vi "Result.Numeric, Compare Value to Limits.vi"(8 "UL":dbl, 9 "LL":dbl, 10 "Value":dbl, 11 "LimType":T2) -> (1 "Desc":string, 3 "Status":T1=3 items=["LOG", "PASS", "FAIL", "ERROR"])   [LabVIEW 2019]
uses:
  Result.Limit Type.ctl
  Result.Measurement and Attribute Item Status.ctl
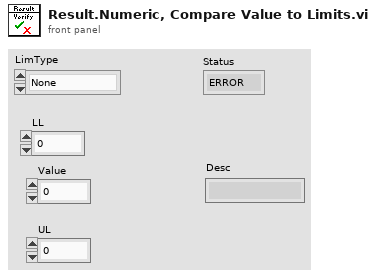
[diagram p1: front panel]
types:
  T1 = typedef "Result.Measurement and Attribute Item Status.ctl" = i32
  T2 = typedef "Result.Limit Type.ctl" = enum16{"None", "EQ", "NE", "GT", "LT", "GE", "LE", "GTLT", "GELE", "GELT", "GTLE", "LTGT", "LEGE", "LEGT", "LTGE", "Contains", "NotContains"}
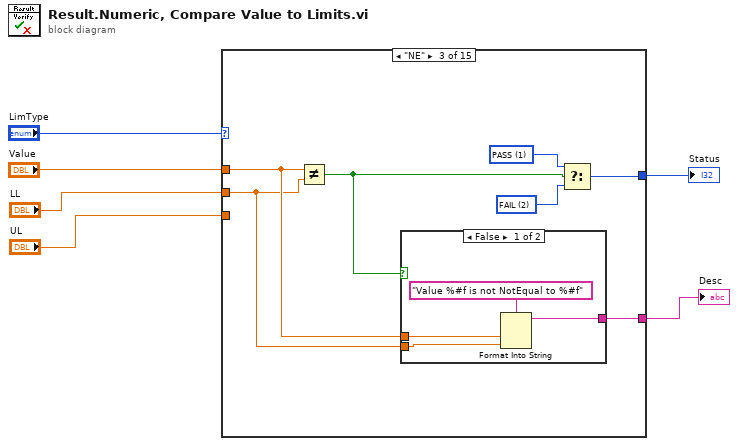
[diagram p0: block diagram]
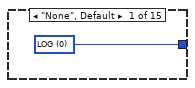
[diagram p2: hidden frame]
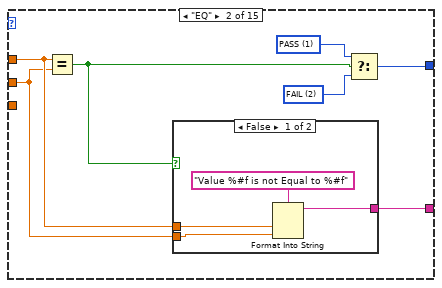
[diagram p3: hidden frame]
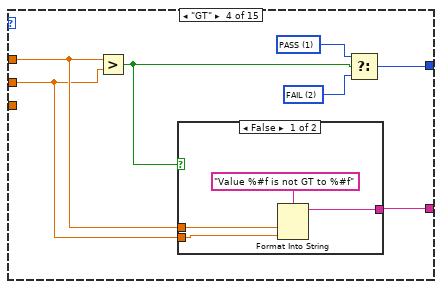
[diagram p6: hidden frame]
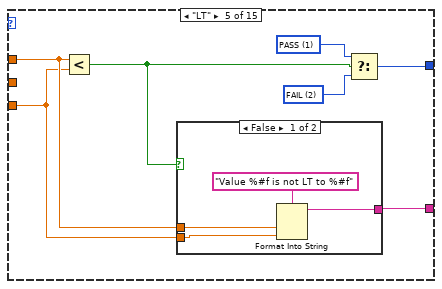
[diagram p8: hidden frame]
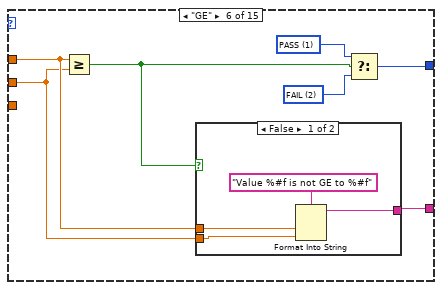
[diagram p10: hidden frame]
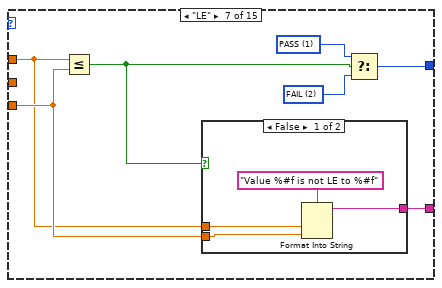
[diagram p12: hidden frame]
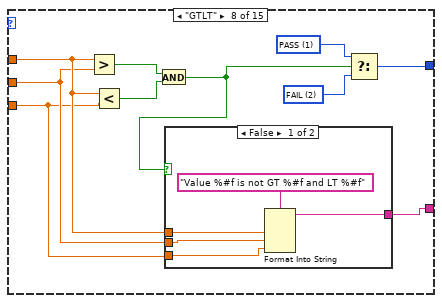
[diagram p14: hidden frame]
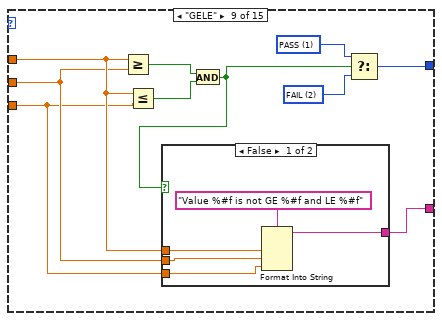
[diagram p16: hidden frame]
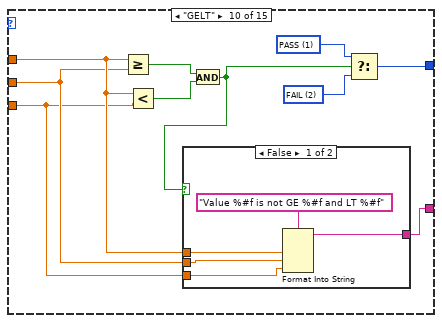
[diagram p18: hidden frame]
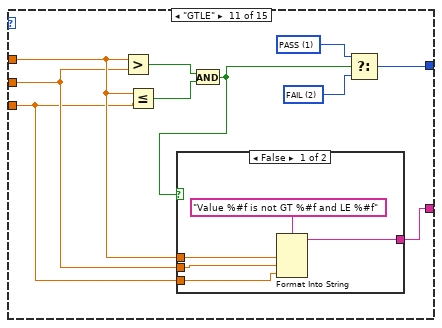
[diagram p20: hidden frame]
diagram:
  n1 = case shown="\"NE\"" "LimType" {
    tunnel: "Value" -> [_ w9 w21 w32 w43 w54 w64 w77 w92 w107 w121 w136 w151 w167 w182]
    tunnel: "LL" -> [_ w8 w20 w31 _ w53 _ w75 w91 w106 w120 w135 w150 w165 w180]
    tunnel: "UL" -> [_ _ _ _ w42 _ w65 w74 w90 w105 w119 w134 w149 w164 w179]
    tunnel: [w7 w14 w25 w36 w47 w58 w69 w83 w98 w113 w128 w143 w158 w173 w188] -> w2
    tunnel: [_ w10 w22 w33 w44 w55 w66 w78 w89 w108 w123 w138 w153 w168 w183] -> w1
    frame "None", Default {
      w7 = T1 0 items=["LOG", "PASS", "FAIL", "ERROR"] ("Status")
    }
    frame "EQ" {
      w12 = T1 2 items=["LOG", "PASS", "FAIL", "ERROR"] ("Status")
      w13 = T1 1 items=["LOG", "PASS", "FAIL", "ERROR"] ("Status")
      n2 = Equal?(x=w9, y=w8) -> (x = y?=w11:bool)
      n3 = case shown="False" w11 {
        tunnel: [w17 _] -> w10
        tunnel: w9 -> [w16 _]
        tunnel: w8 -> [w15 _]
        frame False {
          n4 = Format Into String(format string="Value %#f is not Equal to %#f", w16, w15) -> (resulting string=w17:string)  [unwired: 2 in, 1 out]
        }
        frame True {
        }
      }
      n5 = Select(t=w13, s=w11, f=w12) -> (s? t:f=w14:T1)
    }
    frame "NE" {
      w23 = T1 2 items=["LOG", "PASS", "FAIL", "ERROR"] ("Status")
      w24 = T1 1 items=["LOG", "PASS", "FAIL", "ERROR"] ("Status")
      n6 = Not Equal?(x=w21, y=w20) -> (x != y?=w19:bool)
      n7 = case shown="False" w19 {
        tunnel: [w28 _] -> w22
        tunnel: w21 -> [w27 _]
        tunnel: w20 -> [w26 _]
        frame False {
          n8 = Format Into String(format string="Value %#f is not NotEqual to %#f", w27, w26) -> (resulting string=w28:string)  [unwired: 2 in, 1 out]
        }
        frame True {
        }
      }
      n9 = Select(t=w24, s=w19, f=w23) -> (s? t:f=w25:T1)
    }
    frame "GT" {
      w34 = T1 2 items=["LOG", "PASS", "FAIL", "ERROR"] ("Status")
      w35 = T1 1 items=["LOG", "PASS", "FAIL", "ERROR"] ("Status")
      n10 = Greater?(x=w32, y=w31) -> (0:w30:bool)
      n11 = case shown="False" w30 {
        tunnel: [w39 _] -> w33
        tunnel: w32 -> [w38 _]
        tunnel: w31 -> [w37 _]
        frame False {
          n12 = Format Into String(format string="Value %#f is not GT to %#f", w38, w37) -> (resulting string=w39:string)  [unwired: 2 in, 1 out]
        }
        frame True {
        }
      }
      n13 = Select(t=w35, s=w30, f=w34) -> (s? t:f=w36:T1)
    }
    frame "LT" {
      w45 = T1 2 items=["LOG", "PASS", "FAIL", "ERROR"] ("Status")
      w46 = T1 1 items=["LOG", "PASS", "FAIL", "ERROR"] ("Status")
      n14 = Less?(x=w43, y=w42) -> (x < y?=w41:bool)
      n15 = case shown="False" w41 {
        tunnel: [w50 _] -> w44
        tunnel: w43 -> [w49 _]
        tunnel: w42 -> [w48 _]
        frame False {
          n16 = Format Into String(format string="Value %#f is not LT to %#f", w49, w48) -> (resulting string=w50:string)  [unwired: 2 in, 1 out]
        }
        frame True {
        }
      }
      n17 = Select(t=w46, s=w41, f=w45) -> (s? t:f=w47:T1)
    }
    frame "GE" {
      w56 = T1 2 items=["LOG", "PASS", "FAIL", "ERROR"] ("Status")
      w57 = T1 1 items=["LOG", "PASS", "FAIL", "ERROR"] ("Status")
      n18 = Greater Or Equal?(x=w54, y=w53) -> (x >= y?=w52:bool)
      n19 = case shown="False" w52 {
        tunnel: [w61 _] -> w55
        tunnel: w54 -> [w60 _]
        tunnel: w53 -> [w59 _]
        frame False {
          n20 = Format Into String(format string="Value %#f is not GE to %#f", w60, w59) -> (resulting string=w61:string)  [unwired: 2 in, 1 out]
        }
        frame True {
        }
      }
      n21 = Select(t=w57, s=w52, f=w56) -> (s? t:f=w58:T1)
    }
    frame "LE" {
      w67 = T1 2 items=["LOG", "PASS", "FAIL", "ERROR"] ("Status")
      w68 = T1 1 items=["LOG", "PASS", "FAIL", "ERROR"] ("Status")
      n22 = Less Or Equal?(x=w64, y=w65) -> (x <= y?=w63:bool)
      n23 = case shown="False" w63 {
        tunnel: [w72 _] -> w66
        tunnel: w64 -> [w71 _]
        tunnel: w65 -> [w70 _]
        frame False {
          n24 = Format Into String(format string="Value %#f is not LE to %#f", w71, w70) -> (resulting string=w72:string)  [unwired: 2 in, 1 out]
        }
        frame True {
        }
      }
      n25 = Select(t=w68, s=w63, f=w67) -> (s? t:f=w69:T1)
    }
    frame "GTLT" {
      w81 = T1 2 items=["LOG", "PASS", "FAIL", "ERROR"] ("Status")
      w82 = T1 1 items=["LOG", "PASS", "FAIL", "ERROR"] ("Status")
      n26 = Greater?(x=w77, y=w75) -> (0:w80:bool)
      n27 = Less?(x=w77, y=w74) -> (x < y?=w79:bool)
      n28 = And(x=w80, y=w79) -> (x .and. y?=w76:bool)
      n29 = case shown="False" w76 {
        tunnel: [w87 _] -> w78
        tunnel: w77 -> [w86 _]
        tunnel: w75 -> [w85 _]
        tunnel: w74 -> [w84 _]
        frame False {
          n30 = Format Into String(format string="Value %#f is not GT %#f and LT %#f", w86, w85, w84) -> (resulting string=w87:string)  [unwired: 2 in, 1 out]
        }
        frame True {
        }
      }
      n31 = Select(t=w82, s=w76, f=w81) -> (s? t:f=w83:T1)
    }
    frame "GELE" {
      w96 = T1 2 items=["LOG", "PASS", "FAIL", "ERROR"] ("Status")
      w97 = T1 1 items=["LOG", "PASS", "FAIL", "ERROR"] ("Status")
      n32 = Greater Or Equal?(x=w92, y=w91) -> (x >= y?=w95:bool)
      n33 = Less Or Equal?(x=w92, y=w90) -> (x <= y?=w94:bool)
      n34 = And(x=w95, y=w94) -> (x .and. y?=w93:bool)
      n35 = case shown="False" w93 {
        tunnel: [w102 _] -> w89
        tunnel: w92 -> [w101 _]
        tunnel: w91 -> [w100 _]
        tunnel: w90 -> [w99 _]
        frame False {
          n36 = Format Into String(format string="Value %#f is not GE %#f and LE %#f", w101, w100, w99) -> (resulting string=w102:string)  [unwired: 2 in, 1 out]
        }
        frame True {
        }
      }
      n37 = Select(t=w97, s=w93, f=w96) -> (s? t:f=w98:T1)
    }
    frame "GELT" {
      w111 = T1 2 items=["LOG", "PASS", "FAIL", "ERROR"] ("Status")
      w112 = T1 1 items=["LOG", "PASS", "FAIL", "ERROR"] ("Status")
      n38 = Greater Or Equal?(x=w107, y=w106) -> (x >= y?=w110:bool)
      n39 = Less?(x=w107, y=w105) -> (x < y?=w109:bool)
      n40 = And(x=w110, y=w109) -> (x .and. y?=w104:bool)
      n41 = case shown="False" w104 {
        tunnel: [w117 _] -> w108
        tunnel: w107 -> [w116 _]
        tunnel: w106 -> [w115 _]
        tunnel: w105 -> [w114 _]
        frame False {
          n42 = Format Into String(format string="Value %#f is not GE %#f and LT %#f", w116, w115, w114) -> (resulting string=w117:string)  [unwired: 2 in, 1 out]
        }
        frame True {
        }
      }
      n43 = Select(t=w112, s=w104, f=w111) -> (s? t:f=w113:T1)
    }
    frame "GTLE" {
      w126 = T1 2 items=["LOG", "PASS", "FAIL", "ERROR"] ("Status")
      w127 = T1 1 items=["LOG", "PASS", "FAIL", "ERROR"] ("Status")
      n44 = Greater?(x=w121, y=w120) -> (0:w125:bool)
      n45 = Less Or Equal?(x=w121, y=w119) -> (x <= y?=w124:bool)
      n46 = And(x=w125, y=w124) -> (x .and. y?=w122:bool)
      n47 = case shown="False" w122 {
        tunnel: [w132 _] -> w123
        tunnel: w121 -> [w131 _]
        tunnel: w120 -> [w130 _]
        tunnel: w119 -> [w129 _]
        frame False {
          n48 = Format Into String(format string="Value %#f is not GT %#f and LE %#f", w131, w130, w129) -> (resulting string=w132:string)  [unwired: 2 in, 1 out]
        }
        frame True {
        }
      }
      n49 = Select(t=w127, s=w122, f=w126) -> (s? t:f=w128:T1)
    }
    frame "LTGT" {
      w141 = T1 2 items=["LOG", "PASS", "FAIL", "ERROR"] ("Status")
      w142 = T1 1 items=["LOG", "PASS", "FAIL", "ERROR"] ("Status")
      n50 = Less?(x=w136, y=w135) -> (x < y?=w140:bool)
      n51 = Greater?(x=w136, y=w134) -> (0:w139:bool)
      n52 = Or(x=w140, y=w139) -> (x .or. y?=w137:bool)
      n53 = case shown="False" w137 {
        tunnel: [w147 _] -> w138
        tunnel: w136 -> [w146 _]
        tunnel: w135 -> [w145 _]
        tunnel: w134 -> [w144 _]
        frame False {
          n54 = Format Into String(format string="Value %#f is not LT %#f or GT %#f", w146, w145, w144) -> (resulting string=w147:string)  [unwired: 2 in, 1 out]
        }
        frame True {
        }
      }
      n55 = Select(t=w142, s=w137, f=w141) -> (s? t:f=w143:T1)
    }
    frame "LEGE" {
      w156 = T1 2 items=["LOG", "PASS", "FAIL", "ERROR"] ("Status")
      w157 = T1 1 items=["LOG", "PASS", "FAIL", "ERROR"] ("Status")
      n56 = Less Or Equal?(x=w151, y=w150) -> (x <= y?=w155:bool)
      n57 = Greater Or Equal?(x=w151, y=w149) -> (x >= y?=w154:bool)
      n58 = Or(x=w155, y=w154) -> (x .or. y?=w152:bool)
      n59 = case shown="False" w152 {
        tunnel: [w162 _] -> w153
        tunnel: w151 -> [w161 _]
        tunnel: w150 -> [w160 _]
        tunnel: w149 -> [w159 _]
        frame False {
          n60 = Format Into String(format string="Value %#f is not LE %#f or GE %#f", w161, w160, w159) -> (resulting string=w162:string)  [unwired: 2 in, 1 out]
        }
        frame True {
        }
      }
      n61 = Select(t=w157, s=w152, f=w156) -> (s? t:f=w158:T1)
    }
    frame "LEGT" {
      w171 = T1 2 items=["LOG", "PASS", "FAIL", "ERROR"] ("Status")
      w172 = T1 1 items=["LOG", "PASS", "FAIL", "ERROR"] ("Status")
      n62 = Less Or Equal?(x=w167, y=w165) -> (x <= y?=w170:bool)
      n63 = Greater?(x=w167, y=w164) -> (0:w169:bool)
      n64 = Or(x=w170, y=w169) -> (x .or. y?=w166:bool)
      n65 = case shown="False" w166 {
        tunnel: [w177 _] -> w168
        tunnel: w167 -> [w176 _]
        tunnel: w165 -> [w175 _]
        tunnel: w164 -> [w174 _]
        frame False {
          n66 = Format Into String(format string="Value %#f is not LE %#f or GT %#f", w176, w175, w174) -> (resulting string=w177:string)  [unwired: 2 in, 1 out]
        }
        frame True {
        }
      }
      n67 = Select(t=w172, s=w166, f=w171) -> (s? t:f=w173:T1)
    }
    frame "LTGE" {
      w186 = T1 2 items=["LOG", "PASS", "FAIL", "ERROR"] ("Status")
      w187 = T1 1 items=["LOG", "PASS", "FAIL", "ERROR"] ("Status")
      n68 = Less?(x=w182, y=w180) -> (x < y?=w185:bool)
      n69 = Greater Or Equal?(x=w182, y=w179) -> (x >= y?=w184:bool)
      n70 = Or(x=w185, y=w184) -> (x .or. y?=w181:bool)
      n71 = case shown="False" w181 {
        tunnel: [w192 _] -> w183
        tunnel: w182 -> [w191 _]
        tunnel: w180 -> [w190 _]
        tunnel: w179 -> [w189 _]
        frame False {
          n72 = Format Into String(format string="Value %#f is not LT %#f or GE %#f", w191, w190, w189) -> (resulting string=w192:string)  [unwired: 2 in, 1 out]
        }
        frame True {
        }
      }
      n73 = Select(t=w187, s=w181, f=w186) -> (s? t:f=w188:T1)
    }
  }
  "Status" <- w2
  "Desc" <- w1
